vi "S2C_FORNAX_Poly_EnergyParameterCommand.vi"(8 "Error In":errorcluster, 10 "EnergyParameterCommand":T5={"Partition"="Default", "Message"="EnergyParameterCommand", "M_EnergyChannelId"=0, "M_InstrumentType"=0, "M_ParameterType"=0, "M_EnergyMode"=0, "M_ParameterValue"=0} {"M_EnergyMode" items=["SPRAY_MODE"=0, "CUT_MODE"=1, "BLEND_MODE"=2, "FULGERATE_MODE"=3, "BIPOLAR_MODE"=4, "VESSEL_SEALING_MODE"=5, "VALLEYLAB_MODE"=6, "BIPOLAR_RESECTION_CUT_MODE"=7, "BIPOLAR_RESECTION_COAG_MODE"=8, "AUTOBIPOLAR_MODE"=9, "VIPER_HLA"=10, "SOFT_COAG_MODE"=11, "ECUT_MODE"=12, "SHARED_SPRAY_MODE"=13, "SHARED_FULGERATE_MODE"=14, "CARDIO_MONO_MODE"=15, "CARDIO_BIPOLAR_MODE"=16, "BIPOLAR_LOW_MODE"=17, "BIPOLAR_MACRO_MODE"=18, "BIPOLAR_STANDARD_MODE"=19, "BIPOLAR_MEDIUM_MODE"=20, "VL_ENDOSCOPY_MODE"=21, "NUM_ENERGY_MODES"=22, "MODE_NOT_USED"=-1]; "M_ParameterType" items=["POWER_PARAMETER"=0, "CUT_MODALITY_POWER_PARAMETER"=1, "COAG_MODALITY_POWER_PARAMETER"=2, "VL_MODALITY_POWER_PARAMETER"=3, "BY_MODE_POWER_PARAMETER"=4, "VL_ENDO_CUT_MODALITY_POWER_PARAMETER"=5, "VL_ENDO_COAG_MODALITY_POWER_PARAMETER"=6, "VL_ENDO_COAG_ON_CUT_MODALITY_POWER_PARAMETER"=7, "MODE_PARAMETER"=8, "CUT_MODALITY_MODE_PARAMETER"=9, "COAG_MODALITY_MODE_PARAMETER"=10, "VL_ENDO_COAG_MODALITY_MODE_PARAMETER"=11, "VL_ENDO_CUT_INTERVAL_PARAMETER"=12, "VL_ENDO_CUT_DURATION_PARAMETER"=13, "POWER_BAR_PARAMETER"=14, "MAX_ACTIVATION_MSEC_TIME_PARAMETER"=15, "AUTOBIPOLAR_DELAY_MSEC_TIME"=16, "VL_ENDO_COAG_QUICK_ACCESS_PARAMETER"=17, "PARAMETER_TYPE_NOT_USED"=-1]; "M_InstrumentType" items=["INSTRUMENT_TYPE_UNKNOWN", "INSTRUMENT_TYPE_MONOPOLAR", "INSTRUMENT_TYPE_BIPOLAR", "INSTRUMENT_TYPE_TRIVERSE", "INSTRUMENT_TYPE_LIGASURE", "INSTRUMENT_TYPE_ADVANCE_II", "INSTRUMENT_TYPE_BIPOLAR_RESECTION", "INSTRUMENT_TYPE_HOOK", "INSTRUMENT_TYPE_BIZACT", "INSTRUMENT_TYPE_CARDIOBLATE_BIP", "INSTRUMENT_TYPE_CARDIOBLATE_BIP_GEMINI_S", "INSTRUMENT_TYPE_CARDIOBLATE_MONO", "INSTRUMENT_TYPE_ULTRASONIC", "INSTRUMENT_TYPE_MONOPOLAR_GI", "INSTRUMENT_TYPE_GOLDILOCKS"]; "M_EnergyChannelId" items=["EC_MONO_1"=0, "EC_BIPOLAR"=1, "EC_MONO_2"=2, "EC_ADVANCED"=3, "EC_ADVANCED_ECUT"=4, "EC_ADVANCED_DCUT"=5, "EC_SHARED_COAG"=6, "EC_INTERNAL_BIP_CAL"=7, "EC_NOT_USED"=-1]}, 11 "Settings":T6={"Driver"="Fornax", "Command"="EnergyParameterCommand", "Return"="ErrorStatus", "Parameters"="", "Timeout"=10.0}) -> (0 "Error Out":errorcluster, 3 "Response":string)   [LabVIEW 2015]
uses:
  Typedefs/EnergyChannelId.ctl
  Typedefs/InstrumentType.ctl
  Typedefs/EnergyParameterType.ctl
  Typedefs/EnergyModes.ctl
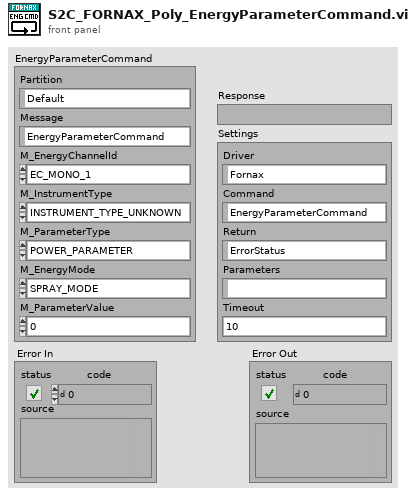
[diagram p1: front panel]
types:
  T1 = typedef "EnergyChannelId.ctl" = i16
  T2 = typedef "InstrumentType.ctl" = i16
  T3 = typedef "EnergyParameterType.ctl" = i16
  T4 = typedef "EnergyModes.ctl" = i16
  T5 = cluster{"Partition":string, "Message":string, "M_EnergyChannelId":T1, "M_InstrumentType":T2, "M_ParameterType":T3, "M_EnergyMode":T4, "M_ParameterValue":i32}
  T6 = cluster{"Driver":string, "Command":string, "Return":string, "Parameters":string, "Timeout":dbl}
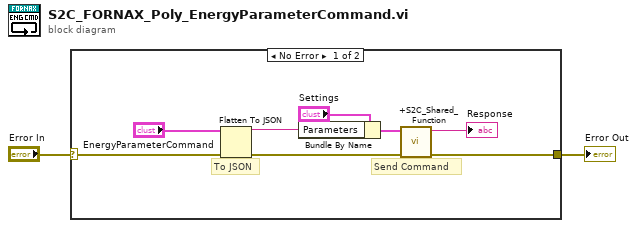
[diagram p0: block diagram]
diagram:
  n1 = case shown="No Error" "Error In" {
    selector: "Error In" -> [w6 w11]
    tunnel: [w5 w11] -> w1
    frame No Error {
      # "To JSON"
      # "Send Command"
      n2 = Flatten To JSON(anything="EnergyParameterCommand", error in (no error)=w6) -> (JSON string=w7:string, 11:w9:errorcluster)  [unwired: 1 in]
      n3 = Bundle By Name(cluster="Settings", "Parameters"=w7) -> (w10:T6)
      n4 = call "+S2C_Shared_Function.vi"("Error In"=w9, "Settings"=w10) -> ("Error Out"=w5:errorcluster, "Response"=→"Response":string)  [unwired: 8 in]
    }
    frame Error {
    }
  }
  "Error Out" <- w1
